vi "Test Clean Source String.vi"(8 "error in (no error)":errorcluster) -> (0 "error out":errorcluster)   [LabVIEW 2016, in "UT_Formatter.lvlib"]
doc: "Template for an unit test with caraya in the \"Given, When, Then\" structure from James."
uses:
  UT_Formatter.lvlib
  Source/HSE-Logger/LogLevel.ctl
  <vilib>/addons/_JKI Toolkits/Caraya/classes/Assert/Assert Equal Value_Variant.vi
  Source/HSE-Logger/Formatter/Formatter.lvclass
  <vilib>/addons/_JKI Toolkits/Caraya/classes/Test/Test.lvclass
  <vilib>/addons/_JKI Toolkits/Caraya/classes/Assert/Assert.lvclass
  Source/HSE-Logger/LogRecord/LogRecord.lvclass
  Source/HSE-Logger/hse-logger.lvlib
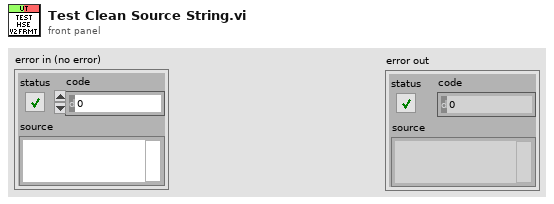
[diagram p1: front panel]
types:
  T1 = typedef "hse-logger.lvlib/LogLevel.ctl" = enum16{"DEBUG", "INFO", "WARNING", "ERROR", "CRITICAL"}
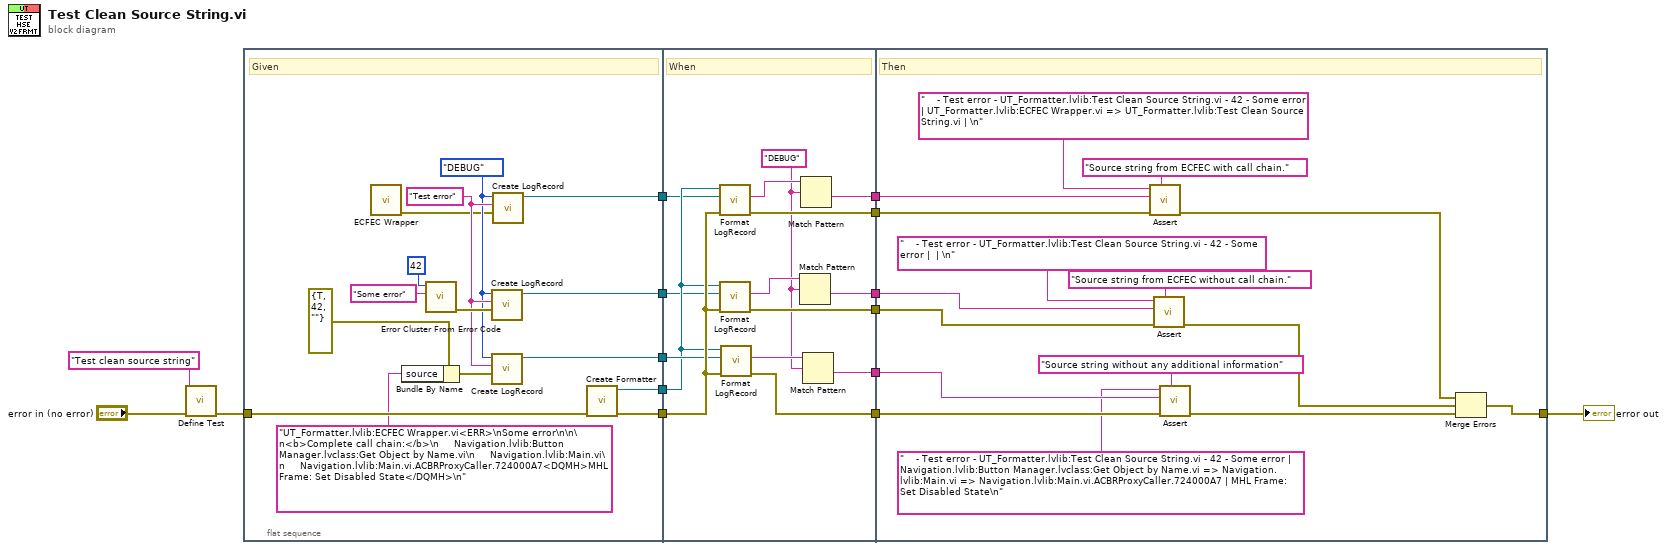
[diagram p0: block diagram]
diagram:
  n1 = call <vilib>:"Define Test.vi"("error in (no error)"="error in (no error)", "Label (VI Title)"="Test clean source string") -> ("error out"=w13:errorcluster)  [unwired: 8 in, 1 out]
  n2 = flat-sequence {
    tunnel: w13 -> [w25]
    tunnel: [w24] -> w10
    tunnel: [w23] -> w9
    tunnel: [w22] -> w8
    tunnel: [w21] -> w7
    tunnel: [w20] -> w6
    tunnel: [w43] -> w11
    tunnel: w10 -> [w45]
    tunnel: w9 -> [w42]
    tunnel: w8 -> [w44]
    tunnel: w7 -> [w41]
    tunnel: w6 -> [w40]
    tunnel: [w32] -> w5
    tunnel: [w33] -> w4
    tunnel: [w31] -> w3
    tunnel: [w39] -> w2
    tunnel: [w38] -> w1
    tunnel: [w61] -> w15
    tunnel: w11 -> [w58]
    tunnel: w5 -> [w52]
    tunnel: w4 -> [w51]
    tunnel: w3 -> [w50]
    tunnel: w2 -> [w54]
    tunnel: w1 -> [w53]
    frame #0 {
      w26 = LogLevel."DEBUG" ("Level")
      w27 = "Test error" ("Message")
      # "Given"
      n3 = call "ECFEC Wrapper.vi"() -> ("error out"=w16:errorcluster)  [unwired: 11 in]
      n4 = Bundle By Name(cluster=errorcluster {"status"=TRUE, "code"=42, "source"=""} ("Error to Log"), "source"="UT_Formatter.lvlib:ECFEC Wrapper.vi<ERR>\nSome error\n\n\n<b>Complete call chain:</b>\n     Navigation.lvlib:Button Manager.lvclass:Get Object by Name.vi\n     Navigation.lvlib:Main.vi\n     Navigation.lvlib:Main.vi.ACBRProxyCaller.724000A7<DQMH>MHL Frame: Set Disabled State</DQMH>\n") -> (w18:errorcluster)
      n5 = call <vilib>:"Error Cluster From Error Code.vi"("error message (\"\")"="Some error" ("error message (\"\")"), "error code (0)"=42) -> ("error out"=w28:errorcluster)  [unwired: 7 in]
      n6 = call "Create LogRecord.vi"("Error to Log"=w28, "Message"=w27, "Level"=w26) -> ("LogRecord out"=w21:refnum<class "LogRecord.lvclass">)  [unwired: 7 in, 1 out]
      n7 = call "Create LogRecord.vi"("Error to Log"=w18, "Message"=w27, "Level"=w26) -> ("LogRecord out"=w22:refnum<class "LogRecord.lvclass">)  [unwired: 7 in, 1 out]
      n8 = call "Create LogRecord.vi"("Error to Log"=w16, "Message"=w27, "Level"=w26) -> ("LogRecord out"=w20:refnum<class "LogRecord.lvclass">)  [unwired: 7 in, 1 out]
      n9 = call "Create Formatter.vi"("error in"=w25) -> ("error out"=w24:errorcluster, "Formatter out"=w23:refnum<class "Formatter.lvclass">)  [unwired: 9 in]
    }
    frame #1 {
      w34 = "DEBUG" ("regular expression")
      # "When"
      n10 = call-dynamic "Format LogRecord.vi"("error in"=w45, "LogRecord"=w40, "Formatter in"=w42) -> ("error out"=w38:errorcluster, "LogLine"=w37:string)  [unwired: 7 in]
      n11 = call-dynamic "Format LogRecord.vi"("error in"=w45, "LogRecord"=w41, "Formatter in"=w42) -> ("error out"=w39:errorcluster, "LogLine"=w36:string)  [unwired: 7 in]
      n12 = call-dynamic "Format LogRecord.vi"("error in"=w45, "LogRecord"=w44, "Formatter in"=w42) -> ("error out"=w43:errorcluster, "LogLine"=w35:string)  [unwired: 7 in]
      n13 = Match Pattern(string=w36, regular expression=w34) -> (after substring=w33:string)  [unwired: 1 in, 3 out]
      n14 = Match Pattern(string=w37, regular expression=w34) -> (after substring=w32:string)  [unwired: 1 in, 3 out]
      n15 = Match Pattern(string=w35, regular expression=w34) -> (after substring=w31:string)  [unwired: 1 in, 3 out]
    }
    frame #2 {
      # "Then"
      n16 = call-poly <vilib>:"Assert.vi"("Label"="Source string from ECFEC with call chain.", "error in (no error)"=w53, "Y"=w52, "X"="    - Test error - UT_Formatter.lvlib:Test Clean Source String.vi - 42 - Some error | UT_Formatter.lvlib:ECFEC Wrapper.vi => UT_Formatter.lvlib:Test Clean Source String.vi | \n" ("Label")) -> ("error out"=w56:errorcluster)  [unwired: 6 in, 1 out]
      n17 = call-poly <vilib>:"Assert.vi"("Label"="Source string from ECFEC without call chain.", "error in (no error)"=w54, "Y"=w51, "X"="    - Test error - UT_Formatter.lvlib:Test Clean Source String.vi - 42 - Some error |  | \n" ("Label")) -> ("error out"=w59:errorcluster)  [unwired: 6 in, 1 out]
      n18 = call-poly <vilib>:"Assert.vi"("Label"="Source string without any additional information", "error in (no error)"=w58, "Y"=w50, "X"="    - Test error - UT_Formatter.lvlib:Test Clean Source String.vi - 42 - Some error | Navigation.lvlib:Button Manager.lvclass:Get Object by Name.vi => Navigation.lvlib:Main.vi => Navigation.lvlib:Main.vi.ACBRProxyCaller.724000A7 | MHL Frame: Set Disabled State\n" ("Label")) -> ("error out"=w60:errorcluster)  [unwired: 6 in, 1 out]
      n19 = Merge Errors(w56, w59, w60) -> (w61:errorcluster)
    }
  }
  "error out" <- w15
